vi "Read Write_.vi"(8 "error in (no error)":errorcluster, 11 "Update Write Ringdowns MSG in":refnum<class "Update Write Ringdowns MSG.lvclass">) -> (0 "error out":errorcluster, 2 "Write?":bool, 3 "Update Write Ringdowns MSG out":refnum<class "Update Write Ringdowns MSG.lvclass">)   [LabVIEW 2014, in "eCRDS Library.lvlib" / "Update Write Ringdowns MSG.lvclass"]
uses:
  Update Write Ringdowns MSG.lvclass
  Update Write Ringdowns MSG.lvclass/Update Write Ringdowns MSG.ctl
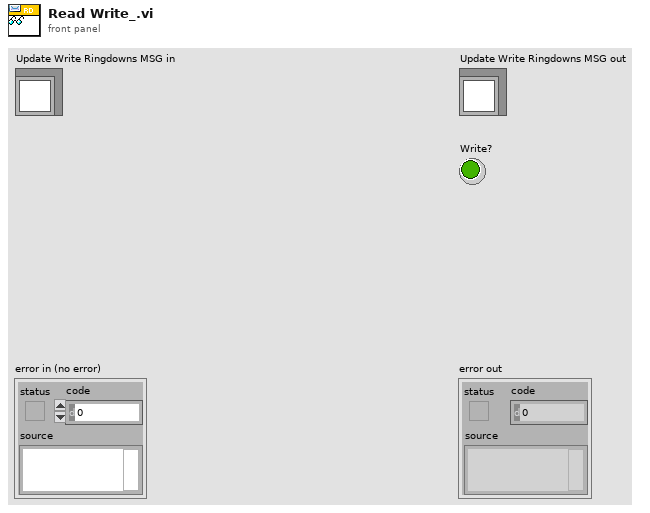
[diagram p1: front panel]
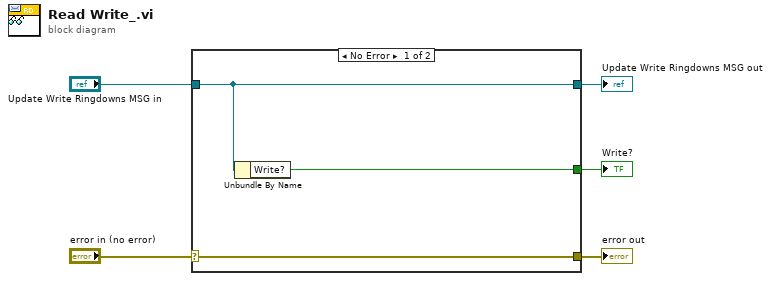
[diagram p0: block diagram]
diagram:
  n1 = case shown="No Error" "error in (no error)" {
    selector: "error in (no error)" -> [w8 w9]
    tunnel: [w8 w9] -> w4
    tunnel: [w7 w10] -> w2
    tunnel: "Update Write Ringdowns MSG in" -> [w7 w10]
    tunnel: [w6 _] -> w1
    frame No Error {
      n2 = Unbundle By Name(w7) -> ("Write?"=w6:bool)
    }
    frame Error {
    }
  }
  "error out" <- w4
  "Update Write Ringdowns MSG out" <- w2
  "Write?" <- w1
